vi "send frame rate.vi"(8 "error in (no error)":errorcluster, 11 "Waveform in":refnum<class "Waveform.lvclass">) -> (0 "error out":errorcluster, 3 "Waveform out":refnum<class "Waveform.lvclass">)   [LabVIEW 2012, in "Waveform.lvclass"]
uses:
  Waveform.lvclass
  Waveform.lvclass/Waveform.ctl
  <vilib>/Distrio/Murmex/Murmex/update_cluster.ctl
  <vilib>/Distrio/Murmex/Murmex/Murmex.lvclass
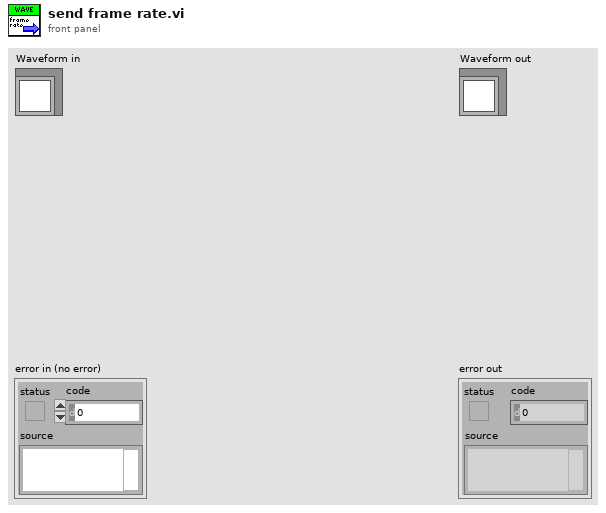
[diagram p1: front panel]
types:
  T1 = typedef "Murmex.lvlib/Murmex.lvclass/update_cluster.ctl" = cluster{"target ID":string, "key chains":string[], "values":variant[]}
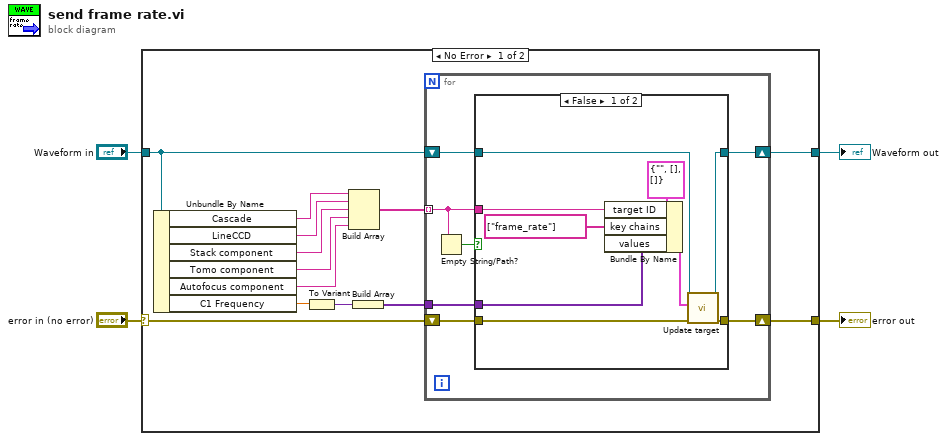
[diagram p0: block diagram]
diagram:
  n1 = case shown="No Error" "error in (no error)" {
    selector: "error in (no error)" -> [w8 w37]
    tunnel: [w7 w37] -> w3
    tunnel: [w9 w36] -> w1
    tunnel: "Waveform in" -> [w10 w36]
    frame No Error {
      n2 = Unbundle By Name(w10) -> ("Cascade"=w17:string, "LineCCD"=w16:string, "Stack component"=w15:string, "Tomo component"=w14:string, "Autofocus component"=w13:string, "C1 Frequency"=w12:dbl)
      n3 = To Variant(anything=w12) -> (Variant=w11:variant)
      n4 = Build Array(w17, w16, w15, w14, w13) -> (w6:string[])
      n5 = Build Array(w11) -> (w5:variant[])
      n6 = for {
        shift-right: [w21] -> w9
        shift-left: w10 -> [w22]
        shift-right: [w23] -> w7
        shift-left: w8 -> [w24]
        tunnel: w6 -> [w19] mode=indexing
        tunnel: w5 -> [w18]
        n7 = Empty String/Path?(string/path=w19) -> (empty?=w20:bool)
        n8 = case shown="False" w20 {
          tunnel: [w32 w34] -> w23
          tunnel: w24 -> [w33 w34]
          tunnel: w22 -> [w30 w35]
          tunnel: [w29 w35] -> w21
          tunnel: w19 -> [w28 _]
          tunnel: w18 -> [w26 _]
          frame False {
            n9 = Bundle By Name(cluster=T1 {"target ID"="", "key chains"=[], "values"=[]} ("update cluster"), "target ID"=w28, "key chains"=string[] ["frame_rate"], "values"=w26) -> (w27:T1)
            n10 = call <vilib>:"Update target.vi"("error in (no error)"=w33, "update cluster"=w27, "MurmexBase in"=w30) -> ("error out"=w32:errorcluster, "MurmexBase out"=w29:refnum<class "Waveform.lvclass">)  [unwired: 7 in]
          }
          frame True {
          }
        }
      }
    }
    frame Error {
    }
  }
  "error out" <- w3
  "Waveform out" <- w1
